vi "Handle Player.vi"(8 "Move Info":T4, 11 "Temp DVR":refnum<data-value>) -> (3 "Temp DVR":refnum<data-value>)   [LabVIEW 2015, in "SB SubVIs.lvlib"]
uses:
  SB SubVIs.lvlib
  Type Defs/Square Cluster.ctl
  Square/Square.lvclass
  Type Defs/Action Enum.ctl
  Type Defs/Direction Enum.ctl
  Type Defs/Status Enum.ctl
  Read-Only Globals.vi
  Globals (private).vi
  Type Defs/SB Type Defs.lvlib
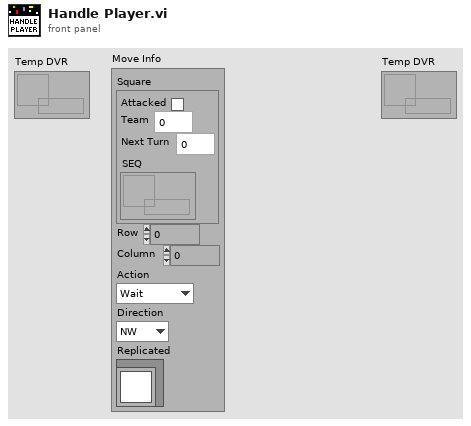
[diagram p1: front panel]
types:
  T1 = typedef "SB Type Defs.lvlib/Square Cluster.ctl" = cluster{"Attacked":bool, "Team":i32, "Next Turn":i32, "SEQ":refnum<queue>}
  T2 = typedef "SB Type Defs.lvlib/Action Enum.ctl" = enum16{"Wait", "Move", "Attack", "Replicate"}
  T3 = typedef "SB Type Defs.lvlib/Direction Enum.ctl" = enum16{"NW", "N", "NE", "E", "SE", "S", "SW", "W"}
  T4 = cluster{"Square":T1, "Row":i32, "Column":i32, "Action":T2, "Direction":T3, "Replicated":refnum<class "Square.lvclass">}
  T5 = typedef "SB Type Defs.lvlib/Status Enum.ctl" = enum16{"Replicate", "Kill", "Eliminate", "Collide"}
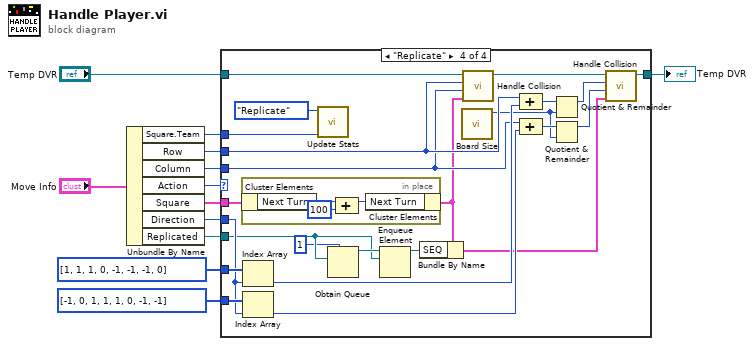
[diagram p0: block diagram]
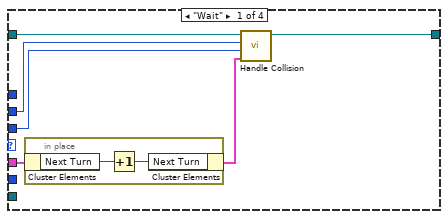
[diagram p2: hidden frame]
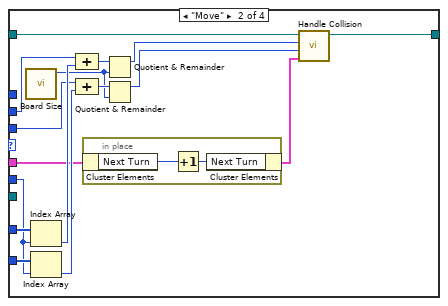
[diagram p3: hidden frame]
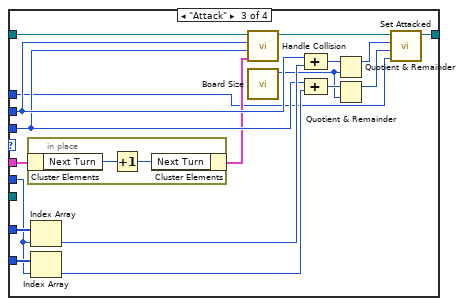
[diagram p4: hidden frame]
diagram:
  n1 = Unbundle By Name("Move Info") -> ("Square.Team"=w1:i32, "Row"=w9:i32, "Column"=w8:i32, "Action"=w12:T2, "Square"=w2:T1, "Direction"=w7:T3, "Replicated"=w6:refnum<class "Square.lvclass">)
  n2 = case shown="\"Replicate\"" w12 {
    tunnel: "Temp DVR" -> [w18 w36 w56 w82]
    tunnel: w9 -> [w17 w30 w48 w74]
    tunnel: w8 -> [w16 w26 w47 w73]
    tunnel: w2 -> [w14 w23 w42 w65]
    tunnel: w7 -> [_ w33 w53 w79]
    tunnel: i32[] [1, 1, 1, 0, -1, -1, -1, 0] -> [_ w35 w55 w81]
    tunnel: i32[] [-1, 0, 1, 1, 1, 0, -1, -1] -> [_ w34 w54 w80]
    tunnel: w6 -> [_ _ _ w61]
    tunnel: [w15 w24 w43 w68] -> w5
    tunnel: w1 -> [_ _ w39 w64]
    frame "Wait" {
      n3 = in-place {
        n4 = in-place-cluster #1(w14) -> ("Next Turn"=w20:i32)
        n5 = Increment(x=w20) -> (x+1=w19:i32)
        n6 = in-place-cluster #1("Next Turn"=w19) -> (w13:T1)
      }
      n7 = call "Handle Collision.vi"("Cluster"=w13, "Column"=w16, "Row"=w17, "Temp DVR"=w18) -> ("Temp DVR"=w15:refnum<data-value>)  [unwired: 7 in]
    }
    frame "Move" {
      n8 = call "Board Size.vi"() -> ("Board Size"=w21:i32)  [unwired: 11 in]
      n9 = Index Array(array=w35, index=w33) -> (element=w29:i32)
      n10 = Index Array(array=w34, index=w33) -> (element=w25:i32)
      n11 = Compound Arithmetic op=ADD(w30, w29) -> (w32:i32)
      n12 = Compound Arithmetic op=ADD(w26, w25) -> (w28:i32)
      n13 = in-place {
        n14 = in-place-cluster #2(w23) -> ("Next Turn"=w38:i32)
        n15 = Increment(x=w38) -> (x+1=w37:i32)
        n16 = in-place-cluster #2("Next Turn"=w37) -> (w22:T1)
      }
      n17 = Quotient & Remainder(x=w32, y=w21) -> (x-y*floor(x/y)=w31:i32)  [unwired: 1 out]
      n18 = Quotient & Remainder(x=w28, y=w21) -> (x-y*floor(x/y)=w27:i32)  [unwired: 1 out]
      n19 = call "Handle Collision.vi"("Cluster"=w22, "Column"=w27, "Row"=w31, "Temp DVR"=w36) -> ("Temp DVR"=w24:refnum<data-value>)  [unwired: 7 in]
    }
    frame "Attack" {
      n20 = in-place {
        n21 = in-place-cluster #3(w42) -> ("Next Turn"=w58:i32)
        n22 = Increment(x=w58) -> (x+1=w57:i32)
        n23 = in-place-cluster #3("Next Turn"=w57) -> (w41:T1)
      }
      n24 = Index Array(array=w55, index=w53) -> (element=w51:i32)
      n25 = Index Array(array=w54, index=w53) -> (element=w49:i32)
      n26 = call "Handle Collision.vi"("Cluster"=w41, "Column"=w47, "Row"=w48, "Temp DVR"=w56) -> ("Temp DVR"=w46:refnum<data-value>)  [unwired: 7 in]
      n27 = call "Board Size.vi"() -> ("Board Size"=w40:i32)  [unwired: 11 in]
      n28 = Compound Arithmetic op=ADD(w48, w51) -> (w52:i32)
      n29 = Compound Arithmetic op=ADD(w47, w49) -> (w50:i32)
      n30 = Quotient & Remainder(x=w52, y=w40) -> (x-y*floor(x/y)=w45:i32)  [unwired: 1 out]
      n31 = Quotient & Remainder(x=w50, y=w40) -> (x-y*floor(x/y)=w44:i32)  [unwired: 1 out]
      n32 = call "Set Attacked.vi"("Team"=w39, "Column"=w44, "Row"=w45, "Temp DVR"=w46) -> ("Temp DVR"=w43:refnum<data-value>)  [unwired: 7 in]
    }
    frame "Replicate" {
      n33 = in-place {
        n34 = in-place-cluster #4(w65) -> ("Next Turn"=w85:i32)
        n35 = Compound Arithmetic op=ADD(w85, 100 ("value")) -> (w84:i32)
        n36 = in-place-cluster #4("Next Turn"=w84) -> (w66:T1)
      }
      n37 = Index Array(array=w81, index=w79) -> (element=w77:i32)
      n38 = Index Array(array=w80, index=w79) -> (element=w75:i32)
      n39 = call "Update Stats.vi"("Team"=w64, "Enum"=Status_Enum."Replicate") -> ()  [unwired: 10 in]
      n40 = Obtain Queue(max queue size (-1, unlimited)=1 ("timeout in ms (-1)"), element data type=w61) -> (queue out=w62:refnum<queue>)  [unwired: 3 in, 2 out]
      n41 = Enqueue Element(queue=w62, element=w61) -> (queue out=w60:refnum<queue>)  [unwired: 2 in, 2 out]
      n42 = Bundle By Name(cluster=w66, "SEQ"=w60) -> (w69:T1)
      n43 = call "Board Size.vi"() -> ("Board Size"=w67:i32)  [unwired: 11 in]
      n44 = call "Handle Collision.vi"("Cluster"=w66, "Column"=w73, "Row"=w74, "Temp DVR"=w82) -> ("Temp DVR"=w72:refnum<data-value>)  [unwired: 7 in]
      n45 = Compound Arithmetic op=ADD(w74, w77) -> (w78:i32)
      n46 = Compound Arithmetic op=ADD(w73, w75) -> (w76:i32)
      n47 = Quotient & Remainder(x=w78, y=w67) -> (x-y*floor(x/y)=w71:i32)  [unwired: 1 out]
      n48 = Quotient & Remainder(x=w76, y=w67) -> (x-y*floor(x/y)=w70:i32)  [unwired: 1 out]
      n49 = call "Handle Collision.vi"("Cluster"=w69, "Column"=w70, "Row"=w71, "Temp DVR"=w72) -> ("Temp DVR"=w68:refnum<data-value>)  [unwired: 7 in]
    }
  }
  "Temp DVR" <- w5
